vi "LVRT Serial Read v1.vi"(6 "Termination Character (Linefeed)":string="\n", 8 "error in (no error)":errorcluster, 9 "Timeout (ms) (-1: no timeout)":i32=-1, 10 "Bytes to Read":u32, 11 "FPGA Main Ref":refnum<k20>) -> (0 "error out":errorcluster, 2 "String":string, 3 "FPGA Main Ref Out":refnum<k20>)   [LabVIEW 2014]
uses:
  <vilib>/rvi/errors/niLvFpgaAdjustHostInterfaceError.vi
  <vilib>/rvi/interface/nirviReadWriteControl/nirviReadWriteControl.xnode
  FPGA Bitfiles/myRIOMidiIn_FPGATarget_FPGAMain_ATizAUb0m2E.lvbitx
  FPGA Main.vi
  NiFpgaLv.dll
panel:
  out "Bytes read so far":u32
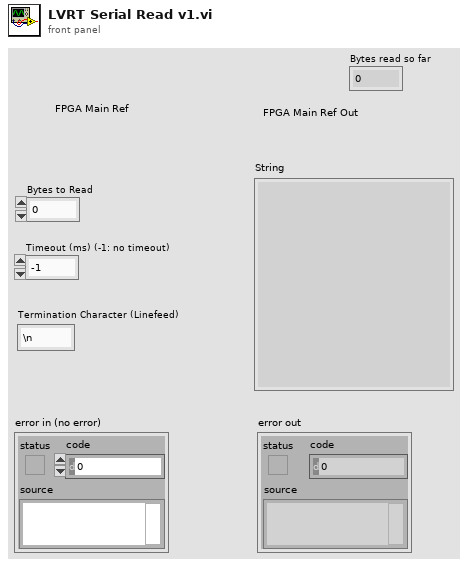
[diagram p1: front panel]
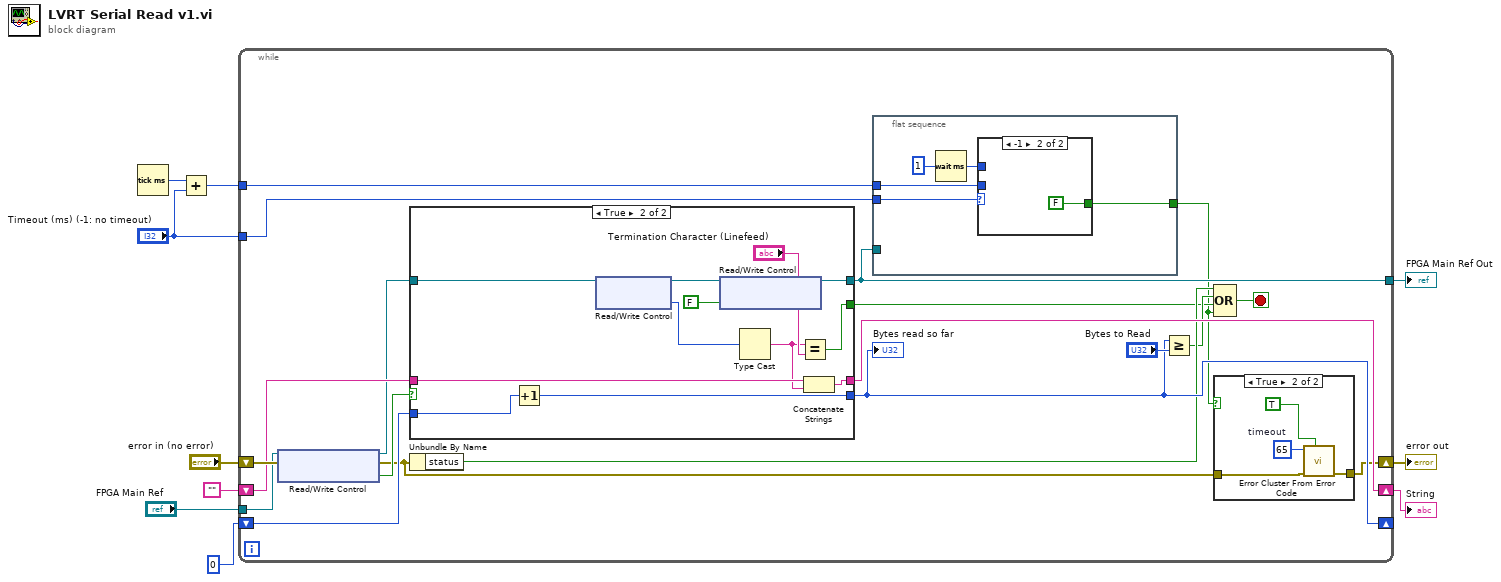
[diagram p0: block diagram]
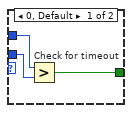
[diagram p3: hidden frame]
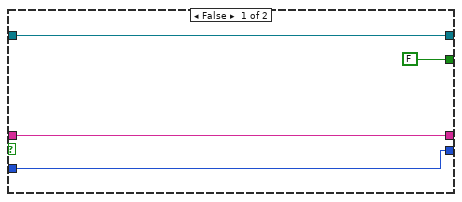
[diagram p4: hidden frame]
diagram:
  n1 = Tick Count (ms)() -> (millisecond timer value=w3:u32)
  n2 = Add(x=w3, y="Timeout (ms) (-1: no timeout)") -> (x+y=w1:u32)
  n3 = while {
    tunnel: "FPGA Main Ref" -> [w23]
    tunnel: [w21] -> w7
    shift-right: [w20] -> _
    shift-left: u32 0 -> [w27]
    shift-right: [w25] -> w4
    shift-left: "" -> [w26]
    shift-right: [w11] -> w9
    shift-left: "error in (no error)" -> [w29]
    tunnel: "Timeout (ms) (-1: no timeout)" -> [w15]
    tunnel: w1 -> [w14]
    stop <- w17 stop-if-true
    n4 = xnode "Read/Write Control"("FPGA VI Reference In"=w23, "error in"=w29) -> ("FPGA VI Reference Out"=w22:refnum<k20>, "error out"=w12:errorcluster, "Read: New Data"=w28:bool)
    n5 = case shown="True" w28 {
      tunnel: [w47 w59] -> w20
      tunnel: w27 -> [w47 w58]
      tunnel: w26 -> [w46 w57]
      tunnel: [w46 w56] -> w25
      tunnel: w22 -> [w45 w54]
      tunnel: [w45 w52] -> w21
      tunnel: [FALSE w48] -> w16
      frame False {
      }
      frame True {
        n6 = Increment(x=w58) -> (x+1=w59:u32)
        n7 = xnode "Read/Write Control"("FPGA VI Reference In"=w54) -> ("FPGA VI Reference Out"=w53:refnum<k20>, "Read: Char"=w55:u8)  [unwired: 1 in, 1 out]
        n8 = xnode "Read/Write Control"("FPGA VI Reference In"=w53, "Read: New Data"=FALSE ("Data Read")) -> ("FPGA VI Reference Out"=w52:refnum<k20>)  [unwired: 1 in, 1 out]
        n9 = Type Cast(x=w55) -> (*(type *) &x=w49:string)  [unwired: 1 out]
        n10 = Equal?(x=w49, y="Termination Character (Linefeed)") -> (x = y?=w48:bool)
        n11 = Concatenate Strings(w57, w49) -> (w56:string)
      }
    }
    "Bytes read so far" <- w20
    n12 = Unbundle By Name(w12) -> ("status"=w19:bool)
    n13 = flat-sequence {
      tunnel: w21 -> [_]
      tunnel: [w38] -> w13
      tunnel: w15 -> [w37]
      tunnel: w14 -> [w36]
      frame #0 {
        n14 = Wait (ms)(milliseconds to wait=u32 1) -> (millisecond timer value=w35:u32)
        n15 = case shown="-1" w37 {
          tunnel: [w40 FALSE] -> w38
          tunnel: w36 -> [w41 _]
          tunnel: w35 -> [w42 _]
          frame 0, Default {
            n16 = Greater? "Check for timeout"(x=w42, y=w41) -> (0:w40:bool)
          }
          frame -1 {
          }
        }
      }
    }
    n17 = Greater Or Equal?(x=w20, y="Bytes to Read") -> (x >= y?=w18:bool)
    n18 = Compound Arithmetic op=OR(w19, w18, w16, w13) -> (w17:bool)
    n19 = case shown="True" w13 {
      tunnel: w12 -> [w30 w34]
      tunnel: [w30 w33] -> w11
      frame False {
      }
      frame True {
        w32 = 65  # timeout
        n20 = call <vilib>:"Error Cluster From Error Code.vi"("show call chain? (False)"=TRUE, "error in (no error)"=w34, "error code (0)"=w32) -> ("error out"=w33:errorcluster)  [unwired: 6 out]
      }
    }
  }
  "error out" <- w9
  "String" <- w4
  "FPGA Main Ref Out" <- w7
